vi "SetServosViaSerial.vi"() -> ()   [LabVIEW 2014]
panel:
  in  "Data":T1(array[cluster])
  in  "VISA resource name":refnum<visa-resource-name>
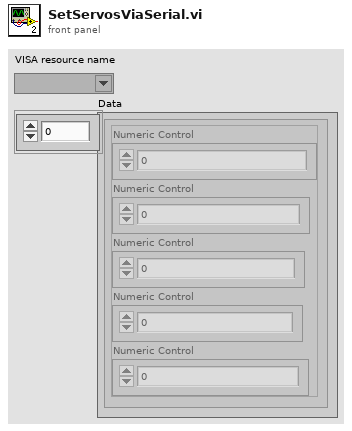
[diagram p1: front panel]
types:
  T1 = cluster{"Numeric Control":dbl, "Numeric Control":dbl, "Numeric Control":dbl, "Numeric Control":dbl, "Numeric Control":dbl}[]
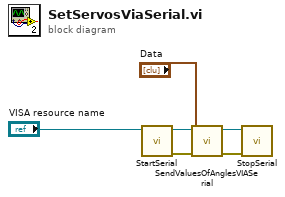
[diagram p0: block diagram]
diagram:
  n1 = call "StartSerial.vi"("VISA Refnum in"="VISA resource name") -> ("error out"=w2:errorcluster, "VISA Refnum out"=w5:refnum<visa-resource-name>)  [unwired: 9 in]
  n2 = call "SendValuesOfAnglesVIASerial.vi"("error in (no error)"=w2, "Data"="Data", "VISA Refnum in"=w5) -> ("error out"=w4:errorcluster, "VISA Refnum out"=w6:refnum<visa-resource-name>)  [unwired: 7 in]
  n3 = call "StopSerial.vi"("error in (no error)"=w4, "VISA Refnum in"=w6) -> ()  [unwired: 10 in]
